vi "read line from table.vi"(8 "error in":errorcluster, 10 "line number":i32, 11 "channels table":T2) -> (0 "error out":errorcluster, 1 "line":T1={"ID"="", "Setpoint"=refnum, "Process Variable"=refnum, "Output"=refnum, "PID gains"={"proportional gain (Kc)"=1.0, "integral time (Ti, min)"=0.01, "derivative time (Td, min)"=0.0}, "output range"={"output high"=100.0, "output low"=-100.0}} {"output range"."output low" format="%.2f"; "output range"."output high" format="%.2f"; "PID gains"."proportional gain (Kc)" format="%.2f"; "PID gains"."integral time (Ti, min)" format="%.2f"}, 2 "empty tag?":bool, 3 "empty channel?":bool)   [LabVIEW 2014, in "Tagbus PID Module editor node.lvclass"]
uses:
  Tagbus PID Module editor node.lvclass
  <vilib>/NI/Tag Bus Module Framework/channel/TBM channel.lvclass
  table reference.ctl
  table line.ctl
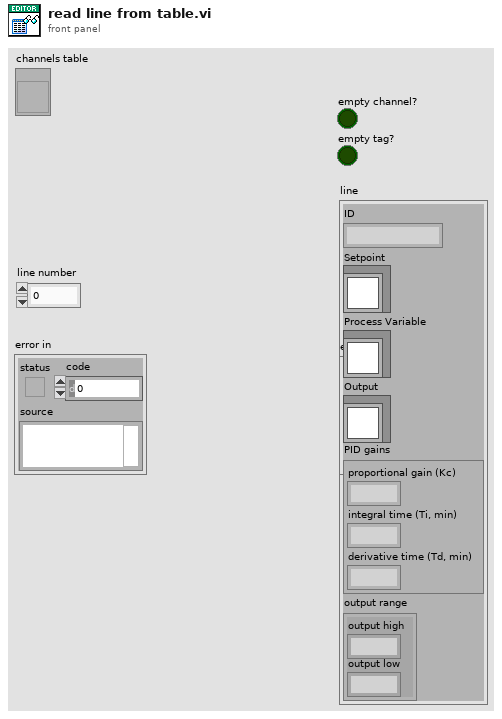
[diagram p1: front panel]
types:
  T1 = typedef "Tagbus PID Module editor node.lvclass/table line.ctl" = cluster{"ID":string, "Setpoint":refnum<class "TBM channel.lvclass">, "Process Variable":refnum<class "TBM channel.lvclass">, "Output":refnum<class "TBM channel.lvclass">, "PID gains":cluster{"proportional gain (Kc)":dbl, "integral time (Ti, min)":dbl, "derivative time (Td, min)":dbl}, "output range":cluster{"output high":dbl, "output low":dbl}}
  T2 = typedef "Tagbus PID Module editor node.lvclass/table reference.ctl" = refnum<vi>
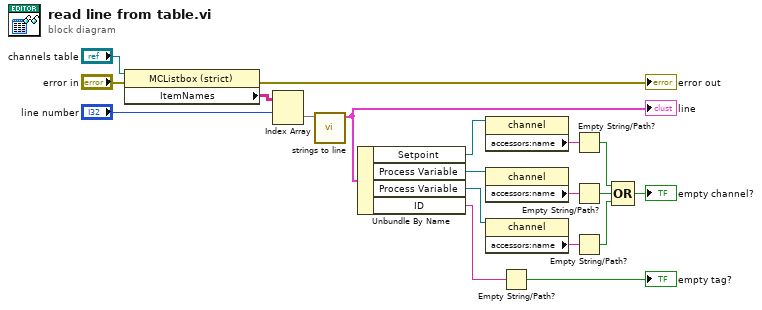
[diagram p0: block diagram]
diagram:
  n1 = property class="MCListbox (strict)"(reference="channels table", error in="error in") -> (error out=→"error out":errorcluster, "ItemNames"=w16:string[][])  [unwired: 1 out]
  n2 = Index Array(array=w16, index (row)="line number") -> (element=w14:string[])  [unwired: 1 in]
  n3 = call "strings to line.vi"("strings"=w14) -> ("line"=w13:T1)  [unwired: 10 in]
  "line" <- w13
  n4 = Unbundle By Name(w13) -> ("Setpoint"=w8:refnum<class "TBM channel.lvclass">, "Process Variable"=w7:refnum<class "TBM channel.lvclass">, "Process Variable"=w12:refnum<class "TBM channel.lvclass">, "ID"=w10:string)
  n5 = property class="channel"(reference=w8) -> ("accessors:name"=w6:string)  [unwired: 1 in, 2 out]
  n6 = property class="channel"(reference=w7) -> ("accessors:name"=w5:string)  [unwired: 1 in, 2 out]
  n7 = property class="channel"(reference=w12) -> ("accessors:name"=w11:string)  [unwired: 1 in, 2 out]
  n8 = Empty String/Path?(string/path=w10) -> (empty?=→"empty tag?":bool)
  n9 = Empty String/Path?(string/path=w6) -> (empty?=w4:bool)
  n10 = Empty String/Path?(string/path=w5) -> (empty?=w3:bool)
  n11 = Empty String/Path?(string/path=w11) -> (empty?=w2:bool)
  n12 = Compound Arithmetic op=OR(w4, w3, w2) -> (→"empty channel?":bool)
